vi "Server.vi"() -> ()   [LabVIEW 2023]
uses:
  <vilib>/OPCUA/controls/Data Type.ctl
  <vilib>/OPCUA/NI OPC UA Server.lvlib
panel:
  in  "Stop Button":bool
  out "Item Node Id":string
  out "Server Endpoint URL":string
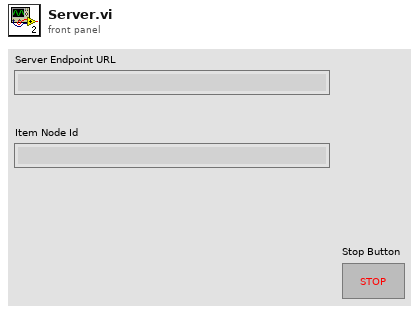
[diagram p1: front panel]
types:
  T1 = typedef "Data Type.ctl" = u16
  T2 = cluster{"name":string, "data type":T1, "access level":u16, "description":string}
  T3 = typedef "OPC UA Server Refnum.ctl" = refnum<k21>
  T4 = typedef "NodeId.ctl" = string
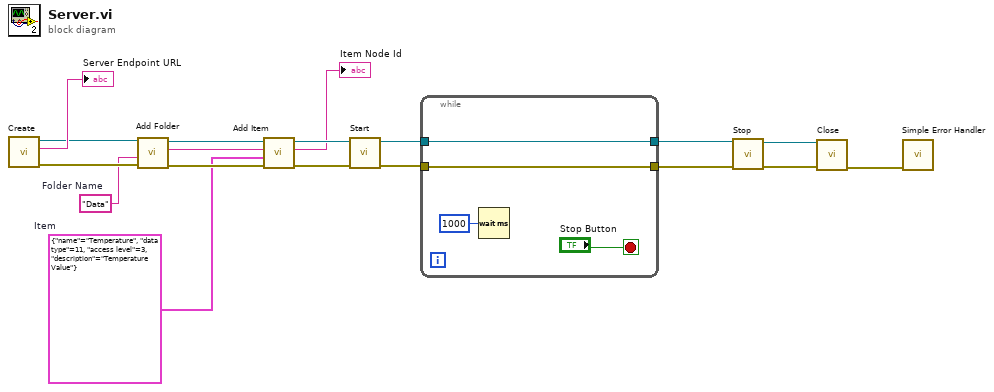
[diagram p0: block diagram]
diagram:
  w6 = T2 {"name"="Temperature", "data type"=11, "access level"=3, "description"="Temperature Value"}  # Item
  w8 = "Data"  # Folder Name
  n1 = call <vilib>:"Create.vi"() -> ("error out"=w17:errorcluster, "server endpoint URL"=→"Server Endpoint URL":string, "OPC UA server refnum out"=w11:T3)  [unwired: 9 in]
  n2 = call <vilib>:"Add Folder.vi"("error in (no error)"=w17, "folder name"=w8, "OPC UA server refnum in"=w11) -> ("error out"=w12:errorcluster, "folder node ID"=w7:T4, "OPC UA server refnum out"=w10:T3)  [unwired: 5 in]
  n3 = call <vilib>:"Add Item.vi"("error in (no error)"=w12, "item"=w6, "parent folder node ID"=w7, "OPC UA server refnum in"=w10) -> ("error out"=w4:errorcluster, "item node ID"=→"Item Node Id":T4, "OPC UA server refnum out"=w5:T3)  [unwired: 3 in, 1 out]
  n4 = call <vilib>:"Start.vi"("error in (no error)"=w4, "OPC UA server refnum in"=w5) -> ("error out"=w3:errorcluster, "OPC UA server refnum out"=w2:T3)  [unwired: 7 in, 1 out]
  n5 = while {
    tunnel: [w20] -> w13
    tunnel: w3 -> [w20]
    tunnel: [w19] -> w9
    tunnel: w2 -> [w19]
    stop <- "Stop Button" stop-if-true
    n6 = Wait (ms)(milliseconds to wait=u32 1000) -> ()  [unwired: 1 out]
  }
  n7 = call <vilib>:"Stop.vi"("error in (no error)"=w13, "OPC UA server refnum in"=w9) -> ("error out"=w14:errorcluster, "OPC UA server refnum out"=w16:T3)  [unwired: 8 in]
  n8 = call <vilib>:"Close.vi"("error in (no error)"=w14, "OPC UA server refnum in"=w16) -> ("error out"=w15:errorcluster)  [unwired: 9 in]
  n9 = call <vilib>:"Simple Error Handler.vi"("error in (no error)"=w15) -> ()  [unwired: 4 in, 5 out]
